vi "Arduino Control.vi"() -> ()   [LabVIEW 2012]
uses:
  <vilib>/Rock Robotics/WPI/DriverStation/WPI_DriverStationAllianceInfo.ctl
  Robot Global Data.vi
  Globals/Useful Values.vi
panel:
  out "Alliance":T1
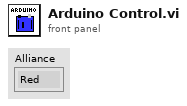
[diagram p1: front panel]
types:
  T1 = typedef "WPI_DriverStationAllianceInfo.ctl" = enum16{"Red", "Blue", "Invalid"}
  T2 = typedef "WPI_DigitalOutputDevRef.ctl" = cluster{"Digital Module":T3, "DIO Channel":T4, "DevStatus":errorcluster}
  T3 = typedef "FPGA_TypedefDigitalModule.ctl" = enum16{"Digital Module 1", "Digital Module 2"}
  T4 = typedef "FPGA_DIOChannel.ctl" = enum8{"DIO 1", "DIO 2", "DIO 3", "DIO 4", "DIO 5", "DIO 6", "DIO 7", "DIO 8", "DIO 9", "DIO 10", "DIO 11", "DIO 12", "DIO 13", "DIO 14", "Invalid"}
  T5 = typedef "WPI_DriverStationRobotMode2.ctl" = enum16{"Autonomous Disabled", "Autonomous Enabled", "Teleop Disabled", "Teleop Enabled", "Timeout", "Finish", "Test Disabled", "Test Enabled"}
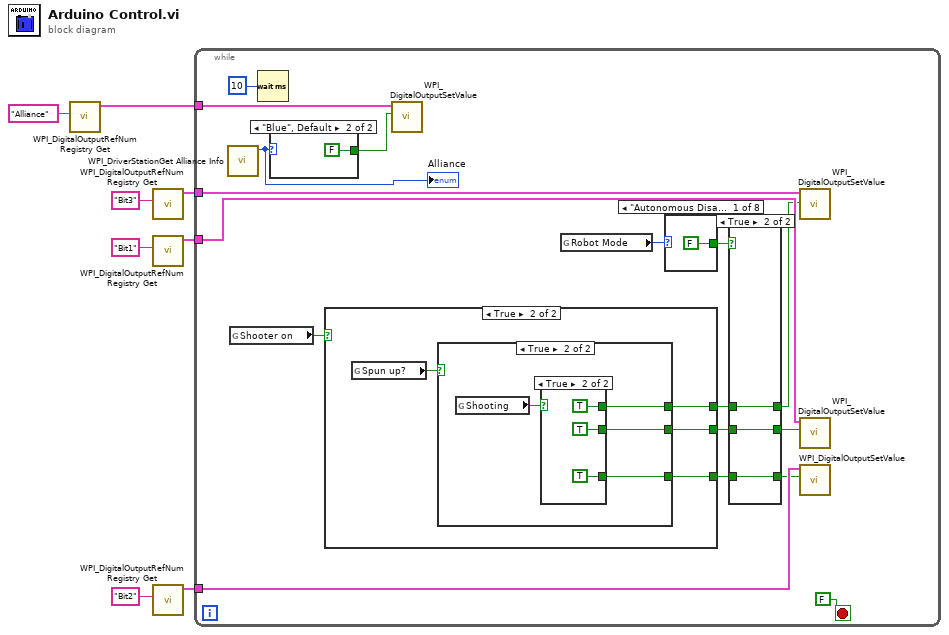
[diagram p0: block diagram]
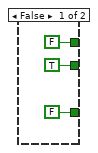
[diagram p2: hidden frame]
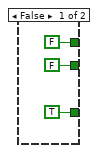
[diagram p3: hidden frame]
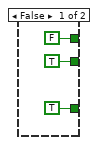
[diagram p4: hidden frame]
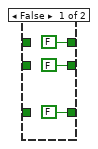
[diagram p5: hidden frame]
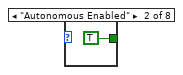
[diagram p6: hidden frame]
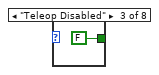
[diagram p7: hidden frame]
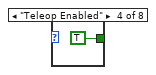
[diagram p8: hidden frame]
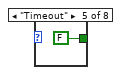
[diagram p9: hidden frame]
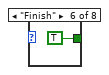
[diagram p10: hidden frame]
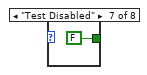
[diagram p11: hidden frame]
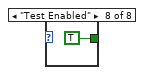
[diagram p12: hidden frame]
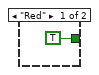
[diagram p13: hidden frame]
diagram:
  n1 = call <vilib>:"WPI_DigitalOutputRefNum Registry Get.vi"("refnum name"="Alliance") -> ("DigitalOutputDevRef"=w7:T2)  [unwired: 9 in, 1 out]
  n2 = call <vilib>:"WPI_DigitalOutputRefNum Registry Get.vi"("refnum name"="Bit3") -> ("DigitalOutputDevRef"=w1:T2)  [unwired: 9 in, 1 out]
  n3 = call <vilib>:"WPI_DigitalOutputRefNum Registry Get.vi"("refnum name"="Bit1") -> ("DigitalOutputDevRef"=w5:T2)  [unwired: 9 in, 1 out]
  n4 = call <vilib>:"WPI_DigitalOutputRefNum Registry Get.vi"("refnum name"="Bit2") -> ("DigitalOutputDevRef"=w4:T2)  [unwired: 9 in, 1 out]
  n5 = while {
    tunnel: w7 -> [w22]
    tunnel: w5 -> [w20]
    tunnel: w4 -> [w19]
    tunnel: w1 -> [w14]
    stop <- FALSE stop-if-true
    n6 = call <vilib>:"WPI_DriverStationGet Alliance Info.vi"() -> ("Alliance"=w23:T1)  [unwired: 10 in, 1 out]
    "Alliance" <- w23
    n7 = global read "Useful Values.vi" "Shooter on"() -> (w12:bool)
    n8 = Wait (ms)(milliseconds to wait=u32 10) -> ()  [unwired: 1 out]
    n9 = case shown="\"Blue\", Default" w23 {
      tunnel: [TRUE FALSE] -> w21
      frame "Red" {
      }
      frame "Blue", Default {
      }
    }
    n10 = case shown="True" w12 {
      tunnel: [TRUE w31] -> w11
      tunnel: [FALSE w30] -> w10
      tunnel: [FALSE w29] -> w9
      frame False {
      }
      frame True {
        n11 = global read "Useful Values.vi" "Spun up?"() -> (w32:bool)
        n12 = case shown="True" w32 {
          tunnel: [FALSE w38] -> w31
          tunnel: [TRUE w37] -> w30
          tunnel: [FALSE w36] -> w29
          frame False {
          }
          frame True {
            n13 = global read "Useful Values.vi" "Shooting"() -> (w39:bool)
            n14 = case shown="True" w39 {
              tunnel: [TRUE TRUE] -> w38
              tunnel: [TRUE TRUE] -> w37
              tunnel: [FALSE TRUE] -> w36
              frame False {
              }
              frame True {
              }
            }
          }
        }
      }
    }
    n15 = call <vilib>:"WPI_DigitalOutputSetValue.vi"("Value"=w21, "DigitalOutputDevRef"=w22) -> ()  [unwired: 8 in, 2 out]
    n16 = global read "Robot Global Data.vi" "Robot Mode"() -> (w18:T5)
    n17 = case shown="\"Autonomous Disabled\", Default" w18 {
      tunnel: [FALSE TRUE FALSE TRUE FALSE TRUE FALSE TRUE] -> w17
      frame "Autonomous Disabled", Default {
      }
      frame "Autonomous Enabled" {
      }
      frame "Teleop Disabled" {
      }
      frame "Teleop Enabled" {
      }
      frame "Timeout" {
      }
      frame "Finish" {
      }
      frame "Test Disabled" {
      }
      frame "Test Enabled" {
      }
    }
    n18 = case shown="True" w17 {
      tunnel: w10 -> [_ w51]
      tunnel: [FALSE w51] -> w16
      tunnel: w11 -> [_ w50]
      tunnel: [FALSE w50] -> w15
      tunnel: [FALSE w49] -> w13
      tunnel: w9 -> [_ w49]
      frame False {
      }
      frame True {
      }
    }
    n19 = call <vilib>:"WPI_DigitalOutputSetValue.vi"("Value"=w13, "DigitalOutputDevRef"=w14) -> ()  [unwired: 8 in, 2 out]
    n20 = call <vilib>:"WPI_DigitalOutputSetValue.vi"("Value"=w15, "DigitalOutputDevRef"=w20) -> ()  [unwired: 8 in, 2 out]
    n21 = call <vilib>:"WPI_DigitalOutputSetValue.vi"("Value"=w16, "DigitalOutputDevRef"=w19) -> ()  [unwired: 8 in, 2 out]
  }
